vi "config.vi"(8 "error in (no error)":errorcluster, 11 "CNT90 in":refnum<class "CNT90.lvclass">) -> (0 "error out":errorcluster, 3 "CNT90 out":refnum<class "CNT90.lvclass">)   [LabVIEW 2019, in "CNT90.lvclass"]
uses:
  CNT90.lvclass
  CNT90.lvclass/CNT90.ctl
  <instrlib>/Pendulum CNT90/Pendulum CNT90.lvlib
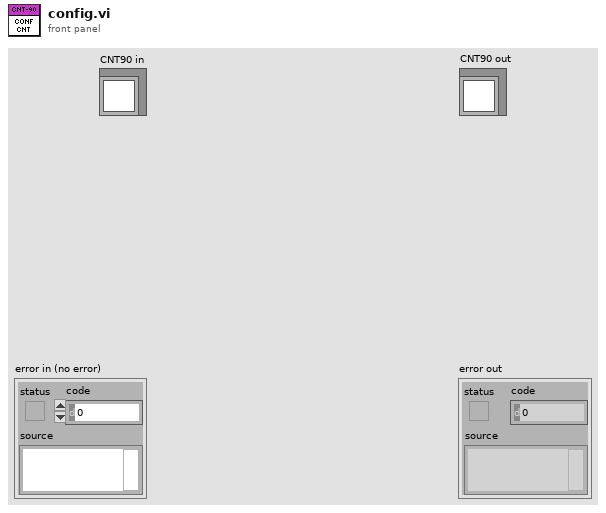
[diagram p1: front panel]
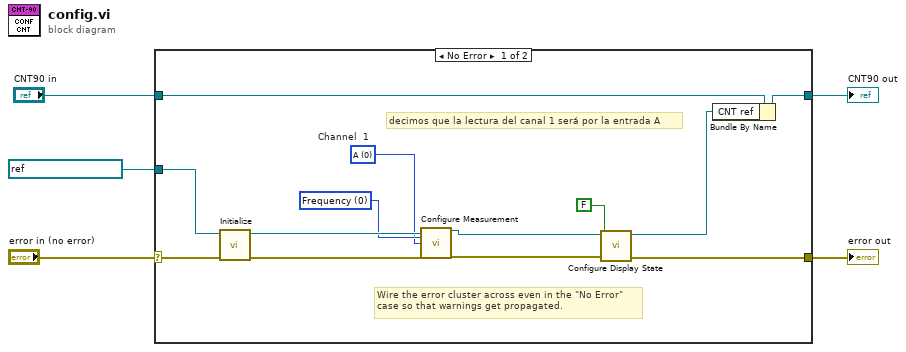
[diagram p0: block diagram]
diagram:
  n1 = case shown="No Error" "error in (no error)" {
    selector: "error in (no error)" -> [w8 w20]
    tunnel: [w9 w20] -> w4
    tunnel: [w7 w19] -> w2
    tunnel: "CNT90 in" -> [w18 w19]
    tunnel: refnum<visa-resource-name> "GPIB0::10::INSTR" ("VISA resource name") -> [w10 _]
    frame No Error {
      w11 = 0 items=["A", "B", "C (HF-input option)", "E (Rear panel arming input)", "A prescaled by 2", "Internal Reference", "A with the variable hysteresis mode"]  # Channel  1
      w14 = 0 items=["Frequency", "Burst Carrier Frequency", "Pulse Repetition Frequency", "Fall-time", "Frequency Ratio", "Positive Peak Voltage", "Negative Peak Voltage", "Negative Pulse Width", "Positive Pulse Width", "Positive Duty Cycle", "Negative Duty Cycle", "Phase", "Period", "Rise-time", "Peak-to-Peak Voltage", "Time-Interval", "Power", "Frequency Back-To-Back", "Period Back-To-Back", "TIE"] ("Measure Function (0: Frequency)")
      # "decimos que la lectura del canal 1 será por la entrada A"
      # "Wire the error cluster across even in the \"No Error\"\ncase so that warnings get propagated."
      n2 = call <instrlib>:"Initialize.vi"("error in (no error)"=w8, "VISA resource name"=w10) -> ("error out"=w17:errorcluster, "VISA resource name out"=w15:refnum<visa-resource-name>)  [unwired: 8 in]
      n3 = call <instrlib>:"Configure Measurement.vi"("VISA resource name"=w15, "Measure Function (0: Frequency)"=w14, "Channel  1 (0: A)"=w11, "error in (no error)"=w17) -> ("VISA resource name out"=w13:refnum<visa-resource-name>, "error out"=w16:errorcluster)  [unwired: 10 in]
      n4 = call <instrlib>:"Configure Display State.vi"("error in (no error)"=w16, "Display State (T: On)"=FALSE, "VISA resource name"=w13) -> ("error out"=w9:errorcluster, "VISA resource name out"=w6:refnum<visa-resource-name>)  [unwired: 7 in]
      n5 = Bundle By Name(cluster=w18, "CNT ref"=w6) -> (w7:refnum<class "CNT90.lvclass">)
    }
    frame Error {
    }
  }
  "error out" <- w4
  "CNT90 out" <- w2
